vi "SubVI_IntializeDrive_Begin.vi"() -> ()   [LabVIEW 2017]
uses:
  <vilib>/Rock Robotics/WPI/SafetyOutput/WPI_SafetyOutputConfigMenu.ctl
  <vilib>/Rock Robotics/WPI/Solenoid/WPI_SolenoidChannel.ctl
  <vilib>/Rock Robotics/WPI/ThirdParty/Phoenix-LabVIEW/Motor Controller/Controls/CTRE_Phoenix_MotorControl_FeedbackDevice.ctl
  <vilib>/Rock Robotics/WPI/Solenoid/WPI_SolenoidOpenSingle.vi
  <vilib>/Rock Robotics/WPI/RobotDrive/WPI_RobotDriveOpen2MotorWithExistingMotors.vi
panel:
  in  "F1":dbl=0.1
  in  "D1":dbl
  in  "I1":dbl
  in  "P1":dbl=0.001
  in  "F0":dbl=0.2
  in  "D0":dbl
  in  "I0":dbl
  in  "P0":dbl=0.001
  in  "secondsFromNeutralToFull":dbl=0.1 format="%#_13g"
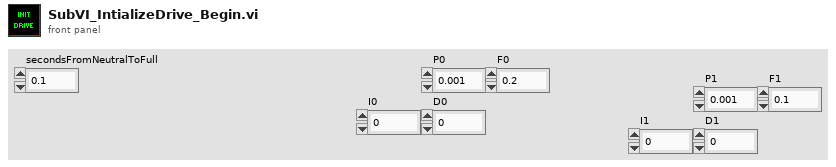
[diagram p1: front panel]
types:
  T1 = typedef "CTRE_Phoenix_MotorControl_FeedbackDevice.ctl" = i8
  T2 = typedef "WPI_SolenoidChannel.ctl" = enum8{"Solenoid 0", "Solenoid 1", "Solenoid 2", "Solenoid 3", "Solenoid 4", "Solenoid 5", "Solenoid 6", "Solenoid 7", "Invalid"}
  T3 = typedef "WPI_SafetyOutputConfigMenu.ctl" = enum16{"Enable", "Disable"}
  T4 = typedef "WPI_SolenoidDevRef.ctl" = cluster{"DevStatus":errorcluster, "Pneumatics Control Module":u8, "Forward Solenoid Channel":T2, "Reverse Solenoid Channel":T2}
  T5 = typedef "WPI_MotorControlDeviceRef.ctl" = cluster{"DeviceStatus":errorcluster, "Type":T6, "PWM":cluster{"PWM Channel":T7, "DeadBand":T8}, "CAN":cluster{"Device Number":u8, "SetOutput VI Ref":variant, "GetOutput VI Ref":variant, "Enable VI Ref":variant, "Disable VI Ref":variant, "Data":variant}, "Invert":bool, "DIO PWM":cluster{"PWM \"Enable\" Channel":T7, "DIOChannel":T9, "PWM Rate":dbl}}
  T6 = typedef "WPI_MotorControlType.ctl" = enum16{"PWM", "CAN", "DIO PWM"}
  T7 = typedef "FPGA_DIOPWMChannel.ctl" = enum8{"PWM 0", "PWM 1", "PWM 2", "PWM 3", "PWM 4", "PWM 5", "PWM 6", "PWM 7", "PWM 8", "PWM 9", "PWM MXP 0", "PWM MXP 1", "PWM MXP 2", "PWM MXP 3", "PWM MXP 4", "PWM MXP 5", "PWM MXP 6", "PWM MXP 7", "PWM MXP 8", "PWM MXP 9", "Invalid"}
  T8 = typedef "WPI_PWMDeadband.ctl" = cluster{"Name":string, "maxPositivePwm":i32, "minPositivePwm":i32, "centerPwm":i32, "maxNegativePwm":i32, "minNegativePwm":i32, "angularRange":u16}
  T9 = typedef "FPGA_DIOChannel.ctl" = enum8{"DIO 0", "DIO 1", "DIO 2", "DIO 3", "DIO 4", "DIO 5", "DIO 6", "DIO 7", "DIO 8", "DIO 9", "DIO MXP 0", "DIO MXP 1", "DIO MXP 2", "DIO MXP 3", "DIO MXP 4", "DIO MXP 5", "DIO MXP 6", "DIO MXP 7", "DIO MXP 8", "DIO MXP 9", "DIO MXP 10", "DIO MXP 11", "DIO MXP 12", "DIO MXP 13", "DIO MXP 14", "DIO MXP 15", "SPI Port CS1", "SPI Port CS2", "SPI Port CS3", "SPI Port MISO", "SPI Port MOSI", "Invalid"}
  T10 = typedef "WPI_RobotDriveDevRef.ctl" = cluster{"DevStatus":errorcluster, "Motors[]":T5[], "Square Inputs":bool, "Max Output":dbl}
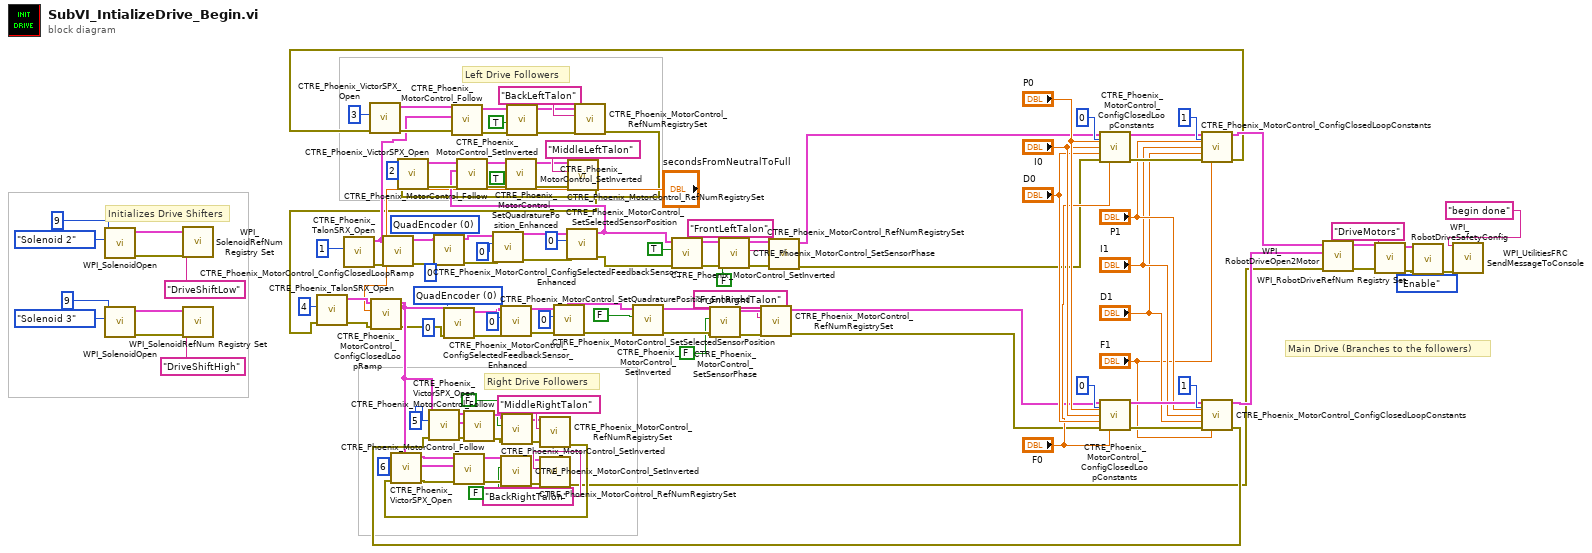
[diagram p0: block diagram]
diagram:
  w4 = T1 0 items=["None"=-1, "QuadEncoder"=0, "Analog"=2, "Tachometer"=4, "Pulse Width Encoded Position"=8, "Sensor Sum (S0 + S1)"=9, "Sensor Difference (D0 - D1)"=10, "Remote Source 0"=11, "Remote Source 1"=12, "Software Emulated"=15] ("Feedback Device")
  w10 = T1 0 items=["None"=-1, "QuadEncoder"=0, "Analog"=2, "Tachometer"=4, "Pulse Width Encoded Position"=8, "Sensor Sum (S0 + S1)"=9, "Sensor Difference (D0 - D1)"=10, "Remote Source 0"=11, "Remote Source 1"=12, "Software Emulated"=15] ("Feedback Device")
  # "Main Drive (Branches to the followers)"
  # "Left Drive Followers"
  # "Initializes Drive Shifters"
  # "Right Drive Followers"
  n1 = call-poly <vilib>:"WPI_SolenoidOpen.vi"("Solenoid Channel"=WPI_SolenoidChannel."Solenoid 2", "Pneumatics Control Module (0)"=u8 9) -> ("error out"=w56:errorcluster, "SolenoidDevRef"=w57:T4)  [unwired: 8 in]
  n2 = call-poly <vilib>:"WPI_SolenoidOpen.vi"("Solenoid Channel"=WPI_SolenoidChannel."Solenoid 3", "Pneumatics Control Module (0)"=u8 9) -> ("error out"=w54:errorcluster, "SolenoidDevRef"=w55:T4)  [unwired: 8 in]
  n3 = call <vilib>:"WPI_SolenoidRefNum Registry Set.vi"("error in (no error)"=w56, "refnum name"="DriveShiftLow", "SolenoidDevRef"=w57) -> ()  [unwired: 7 in, 2 out]
  n4 = call <vilib>:"WPI_SolenoidRefNum Registry Set.vi"("error in (no error)"=w54, "refnum name"="DriveShiftHigh", "SolenoidDevRef"=w55) -> ()  [unwired: 7 in, 2 out]
  n5 = call <vilib>:"CTRE_Phoenix_TalonSRX_Open.vi"("Device Number"=u8 1) -> ("error out"=w47:errorcluster, "CAN Talon SRX Ref"=w46:T5)  [unwired: 9 in]
  n6 = call <vilib>:"CTRE_Phoenix_MotorControl_ConfigClosedLoopRamp.vi"("error in (no error)"=w47, "secondsFromNeutralToFull"="secondsFromNeutralToFull", "PhoenixMotorControlDevRef"=w46) -> ("error out"=w11:errorcluster, "PhoenixMotorControlDevRef"=w12:T5)  [unwired: 7 in]
  n7 = call <vilib>:"CTRE_Phoenix_MotorControl_ConfigSelectedFeedbackSensor_Enhanced.vi"("error in (no error)"=w11, "pidLoopIdx"=0, "Feedback Device"=w10, "PhoenixMotorControlDevRef"=w12) -> ("error out"=w7:errorcluster, "PhoenixMotorControlDevRef"=w8:T5)  [unwired: 6 in]
  n8 = call <vilib>:"CTRE_Phoenix_MotorControl_SetQuadraturePosition_Enhanced.vi"("error in (no error)"=w7, "New Position"=0, "PhoenixMotorControlDevRef"=w8) -> ("error out"=w66:errorcluster, "PhoenixMotorControlDevRef"=w67:T5)  [unwired: 7 in]
  n9 = call <vilib>:"CTRE_Phoenix_MotorControl_SetSelectedSensorPosition.vi"("error in (no error)"=w66, "New Sensor Position"=0, "PhoenixMotorControlDevRef"=w67) -> ("error out"=w64:errorcluster, "PhoenixMotorControlDevRef"=w65:T5)  [unwired: 7 in]
  n10 = call <vilib>:"CTRE_Phoenix_MotorControl_SetInverted.vi"("error in (no error)"=w64, "Invert?"=TRUE, "PhoenixMotorControlDevRef"=w65) -> ("error out"=w122:errorcluster, "PhoenixMotorControlDevRef"=w121:T5)  [unwired: 7 in]
  n11 = call <vilib>:"CTRE_Phoenix_MotorControl_SetSensorPhase.vi"("error in (no error)"=w122, "PhaseSensor"=FALSE, "PhoenixMotorControlDevRef"=w121) -> ("error out"=w117:errorcluster, "PhoenixMotorControlDevRef"=w118:T5)  [unwired: 7 in]
  n12 = call <vilib>:"CTRE_Phoenix_MotorControl_RefNumRegistrySet.vi"("error in (no error)"=w117, "refnum name"="FrontLeftTalon", "PhoenixMotorControlDevRef"=w118) -> ("error out"=w23:errorcluster, "PhoenixMotorControlDevRef"=w26:T5)  [unwired: 7 in]
  n13 = call <vilib>:"CTRE_Phoenix_MotorControl_ConfigClosedLoopConstants.vi"("PhoenixMotorControlDevRef"=w26, "slotIdx"=0, "P"="P0", "I"="I0", "D"="D0", "error in (no error)"=w23, "F"="F0") -> ("PhoenixMotorControlDevRef"=w40:T5, "error out"=w39:errorcluster)  [unwired: 7 in]
  n14 = call <vilib>:"CTRE_Phoenix_MotorControl_ConfigClosedLoopConstants.vi"("PhoenixMotorControlDevRef"=w40, "slotIdx"=1, "P"="P1", "I"="I1", "D"="D1", "error in (no error)"=w39, "F"="F1") -> ("PhoenixMotorControlDevRef"=w22:T5, "error out"=w20:errorcluster)  [unwired: 7 in]
  n15 = call <vilib>:"CTRE_Phoenix_VictorSPX_Open.vi"("error in"=w20, "Device Number"=u8 3) -> ("error out"=w94:errorcluster, "CAN Talon SRX Ref"=w93:T5)  [unwired: 8 in]
  n16 = call <vilib>:"CTRE_Phoenix_MotorControl_Follow.vi"("error in (no error)"=w94, "Master Controller to Follow"=w46, "PhoenixMotorControlDevRef"=w93) -> ("error out"=w76:errorcluster, "PhoenixMotorControlDevRef"=w77:T5)  [unwired: 7 in]
  n17 = call <vilib>:"CTRE_Phoenix_MotorControl_SetInverted.vi"("error in (no error)"=w76, "Invert?"=TRUE, "PhoenixMotorControlDevRef"=w77) -> ("error out"=w74:errorcluster, "PhoenixMotorControlDevRef"=w75:T5)  [unwired: 7 in]
  n18 = call <vilib>:"CTRE_Phoenix_MotorControl_RefNumRegistrySet.vi"("error in (no error)"=w74, "refnum name"="BackLeftTalon", "PhoenixMotorControlDevRef"=w75) -> ("error out"=w19:errorcluster)  [unwired: 7 in, 1 out]
  n19 = call <vilib>:"CTRE_Phoenix_VictorSPX_Open.vi"("error in"=w19, "Device Number"=u8 2) -> ("error out"=w103:errorcluster, "CAN Talon SRX Ref"=w104:T5)  [unwired: 8 in]
  n20 = call <vilib>:"CTRE_Phoenix_MotorControl_Follow.vi"("error in (no error)"=w103, "Master Controller to Follow"=w65, "PhoenixMotorControlDevRef"=w104) -> ("error out"=w82:errorcluster, "PhoenixMotorControlDevRef"=w83:T5)  [unwired: 7 in]
  n21 = call <vilib>:"CTRE_Phoenix_MotorControl_SetInverted.vi"("error in (no error)"=w82, "Invert?"=TRUE, "PhoenixMotorControlDevRef"=w83) -> ("error out"=w80:errorcluster, "PhoenixMotorControlDevRef"=w81:T5)  [unwired: 7 in]
  n22 = call <vilib>:"CTRE_Phoenix_MotorControl_RefNumRegistrySet.vi"("error in (no error)"=w80, "refnum name"="MiddleLeftTalon", "PhoenixMotorControlDevRef"=w81) -> ("error out"=w18:errorcluster)  [unwired: 7 in, 1 out]
  n23 = call <vilib>:"CTRE_Phoenix_TalonSRX_Open.vi"("error in"=w18, "Device Number"=u8 4) -> ("error out"=w44:errorcluster, "CAN Talon SRX Ref"=w45:T5)  [unwired: 8 in]
  n24 = call <vilib>:"CTRE_Phoenix_MotorControl_ConfigClosedLoopRamp.vi"("error in (no error)"=w44, "secondsFromNeutralToFull"="secondsFromNeutralToFull", "PhoenixMotorControlDevRef"=w45) -> ("error out"=w5:errorcluster, "PhoenixMotorControlDevRef"=w6:T5)  [unwired: 7 in]
  n25 = call <vilib>:"CTRE_Phoenix_MotorControl_ConfigSelectedFeedbackSensor_Enhanced.vi"("error in (no error)"=w5, "pidLoopIdx"=0, "Feedback Device"=w4, "PhoenixMotorControlDevRef"=w6) -> ("error out"=w2:errorcluster, "PhoenixMotorControlDevRef"=w1:T5)  [unwired: 6 in]
  n26 = call <vilib>:"CTRE_Phoenix_MotorControl_SetQuadraturePosition_Enhanced.vi"("error in (no error)"=w2, "New Position"=0, "PhoenixMotorControlDevRef"=w1) -> ("error out"=w61:errorcluster, "PhoenixMotorControlDevRef"=w63:T5)  [unwired: 7 in]
  n27 = call <vilib>:"CTRE_Phoenix_MotorControl_SetSelectedSensorPosition.vi"("error in (no error)"=w61, "New Sensor Position"=0, "PhoenixMotorControlDevRef"=w63) -> ("error out"=w60:errorcluster, "PhoenixMotorControlDevRef"=w62:T5)  [unwired: 7 in]
  n28 = call <vilib>:"CTRE_Phoenix_MotorControl_SetInverted.vi"("error in (no error)"=w60, "Invert?"=FALSE, "PhoenixMotorControlDevRef"=w62) -> ("error out"=w124:errorcluster, "PhoenixMotorControlDevRef"=w123:T5)  [unwired: 7 in]
  n29 = call <vilib>:"CTRE_Phoenix_MotorControl_SetSensorPhase.vi"("error in (no error)"=w124, "PhaseSensor"=FALSE, "PhoenixMotorControlDevRef"=w123) -> ("error out"=w116:errorcluster, "PhoenixMotorControlDevRef"=w115:T5)  [unwired: 7 in]
  n30 = call <vilib>:"CTRE_Phoenix_MotorControl_RefNumRegistrySet.vi"("error in (no error)"=w116, "refnum name"="FrontRightTalon", "PhoenixMotorControlDevRef"=w115) -> ("error out"=w24:errorcluster, "PhoenixMotorControlDevRef"=w25:T5)  [unwired: 7 in]
  n31 = call <vilib>:"CTRE_Phoenix_MotorControl_ConfigClosedLoopConstants.vi"("PhoenixMotorControlDevRef"=w25, "slotIdx"=0, "P"="P0", "I"="I0", "D"="D0", "error in (no error)"=w24, "F"="F0") -> ("PhoenixMotorControlDevRef"=w36:T5, "error out"=w35:errorcluster)  [unwired: 7 in]
  n32 = call <vilib>:"CTRE_Phoenix_MotorControl_ConfigClosedLoopConstants.vi"("PhoenixMotorControlDevRef"=w36, "slotIdx"=1, "P"="P1", "I"="I1", "D"="D1", "error in (no error)"=w35, "F"="F1") -> ("PhoenixMotorControlDevRef"=w21:T5, "error out"=w17:errorcluster)  [unwired: 7 in]
  n33 = call <vilib>:"CTRE_Phoenix_VictorSPX_Open.vi"("error in"=w17, "Device Number"=u8 5) -> ("error out"=w101:errorcluster, "CAN Talon SRX Ref"=w102:T5)  [unwired: 8 in]
  n34 = call <vilib>:"CTRE_Phoenix_MotorControl_Follow.vi"("error in (no error)"=w101, "Master Controller to Follow"=w6, "PhoenixMotorControlDevRef"=w102) -> ("error out"=w88:errorcluster, "PhoenixMotorControlDevRef"=w89:T5)  [unwired: 7 in]
  n35 = call <vilib>:"CTRE_Phoenix_MotorControl_SetInverted.vi"("error in (no error)"=w88, "Invert?"=FALSE, "PhoenixMotorControlDevRef"=w89) -> ("error out"=w70:errorcluster, "PhoenixMotorControlDevRef"=w71:T5)  [unwired: 7 in]
  n36 = call <vilib>:"CTRE_Phoenix_MotorControl_RefNumRegistrySet.vi"("error in (no error)"=w70, "refnum name"="MiddleRightTalon", "PhoenixMotorControlDevRef"=w71) -> ("error out"=w16:errorcluster)  [unwired: 7 in, 1 out]
  n37 = call <vilib>:"CTRE_Phoenix_VictorSPX_Open.vi"("error in"=w16, "Device Number"=u8 6) -> ("error out"=w91:errorcluster, "CAN Talon SRX Ref"=w92:T5)  [unwired: 8 in]
  n38 = call <vilib>:"CTRE_Phoenix_MotorControl_Follow.vi"("error in (no error)"=w91, "Master Controller to Follow"=w6, "PhoenixMotorControlDevRef"=w92) -> ("error out"=w86:errorcluster, "PhoenixMotorControlDevRef"=w87:T5)  [unwired: 7 in]
  n39 = call <vilib>:"CTRE_Phoenix_MotorControl_SetInverted.vi"("error in (no error)"=w86, "Invert?"=FALSE, "PhoenixMotorControlDevRef"=w87) -> ("error out"=w72:errorcluster, "PhoenixMotorControlDevRef"=w73:T5)  [unwired: 7 in]
  n40 = call <vilib>:"CTRE_Phoenix_MotorControl_RefNumRegistrySet.vi"("error in (no error)"=w72, "refnum name"="BackRightTalon", "PhoenixMotorControlDevRef"=w73) -> ("error out"=w15:errorcluster)  [unwired: 7 in, 1 out]
  n41 = call-poly <vilib>:"WPI_RobotDriveOpen2Motor.vi"("error in (no error)"=w15, "Right Motor Dev Ref"=w21, "Left Motor Dev Ref"=w22) -> ("error out"=w14:errorcluster, "RobotDriveDevRef"=w109:T10)  [unwired: 7 in]
  n42 = call <vilib>:"WPI_RobotDriveRefNum Registry Set.vi"("error in (no error)"=w14, "refnum name"="DriveMotors", "RobotDriveDevRef"=w109) -> ("error out"=w13:errorcluster, "RobotDriveDevRef"=w112:T10)  [unwired: 7 in]
  n43 = call <vilib>:"WPI_RobotDriveSafetyConfig.vi"("error in (no error)"=w13, "mode"=WPI_SafetyOutputConfigMenu."Enable", "RobotDriveDevRef"=w112) -> ("error out"=w126:errorcluster)  [unwired: 7 in, 1 out]
  n44 = call <vilib>:"WPI_UtilitiesFRC SendMessageToConsole.vi"("Message"="begin done", "error in (no error)"=w126) -> ()  [unwired: 13 in, 1 out]
